vi "Init.vi"(0 "FrontPanelData in":refnum<class "EpiWrapper.lvclass">, 1 "MeasureControl":refnum<vi>, 3 "SpectrumSat":refnum<vi>, 4 "Configuration":refnum<vi>, 5 "WaferTable_Ref":refnum<vi>, 7 "error in (no error)":errorcluster, 8 "MapPositions":refnum<vi>, 9 "WaferMao":refnum<vi>, 11 "CurrentPad":refnum<vi>, 12 "Input":refnum<vi>, 13 "WaferPads":refnum<vi>, 15 "IntTime_Ref":refnum<vi>, 16 "AppPaths":refnum<vi>, 17 "INSTR_PARAM":refnum<vi>) -> (20 "FrontPanelData out":refnum<class "EpiWrapper.lvclass">, 21 "Shutdown?":bool, 27 "error out":errorcluster)   [LabVIEW 2012, in "EpiWrapper.lvclass"]
uses:
  EpiWrapper.lvclass
  Controls/Instr_Param.ctl
  Instruments/TypeDefs/SMUParam.ctl
  Controls/USB4000_Data.ctl
  Controls/WaferTable.ctl
  Controls/Config.ctl
  Controls/SelectedPads.ctl
  Controls/Pad.ctl
  Controls/MeasureControl.ctl
  Controls/PadArea.ctl
  Controls/TestData.ctl
  Controls/Measurement.ctl
  EpiWrapper.lvclass/EpiWrapper.ctl
  Instruments.lvclass
  Controls/ProbeStationId.vi
  LotData.lvclass
panel:
  # "Measure Control"
  # "Measurement Settings"
  # "Test Criteria"
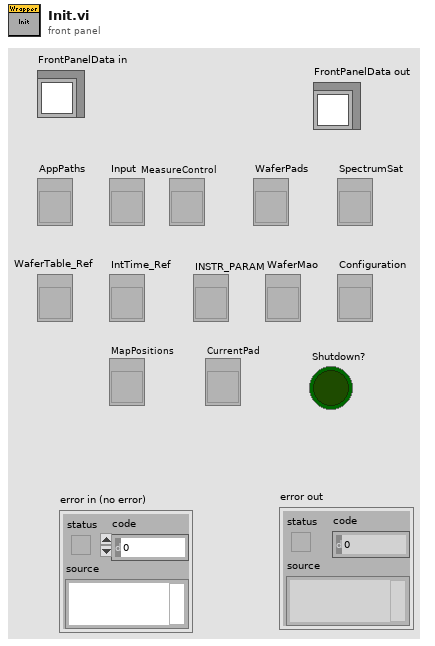
[diagram p1: front panel]
types:
  T1 = typedef "ErrorActions.ctl" = enum16{"Shutdown", "Warning", "Reset", "NoAction"}
  T2 = typedef "Config.ctl" = cluster{"IntTime":i32, "Samples":i32, "PowerMin":dbl, "KneeMin":dbl, "KneeMax":dbl, "Background Wl":dbl, "Settle Delay,ms":u32, "StationId":sgl}
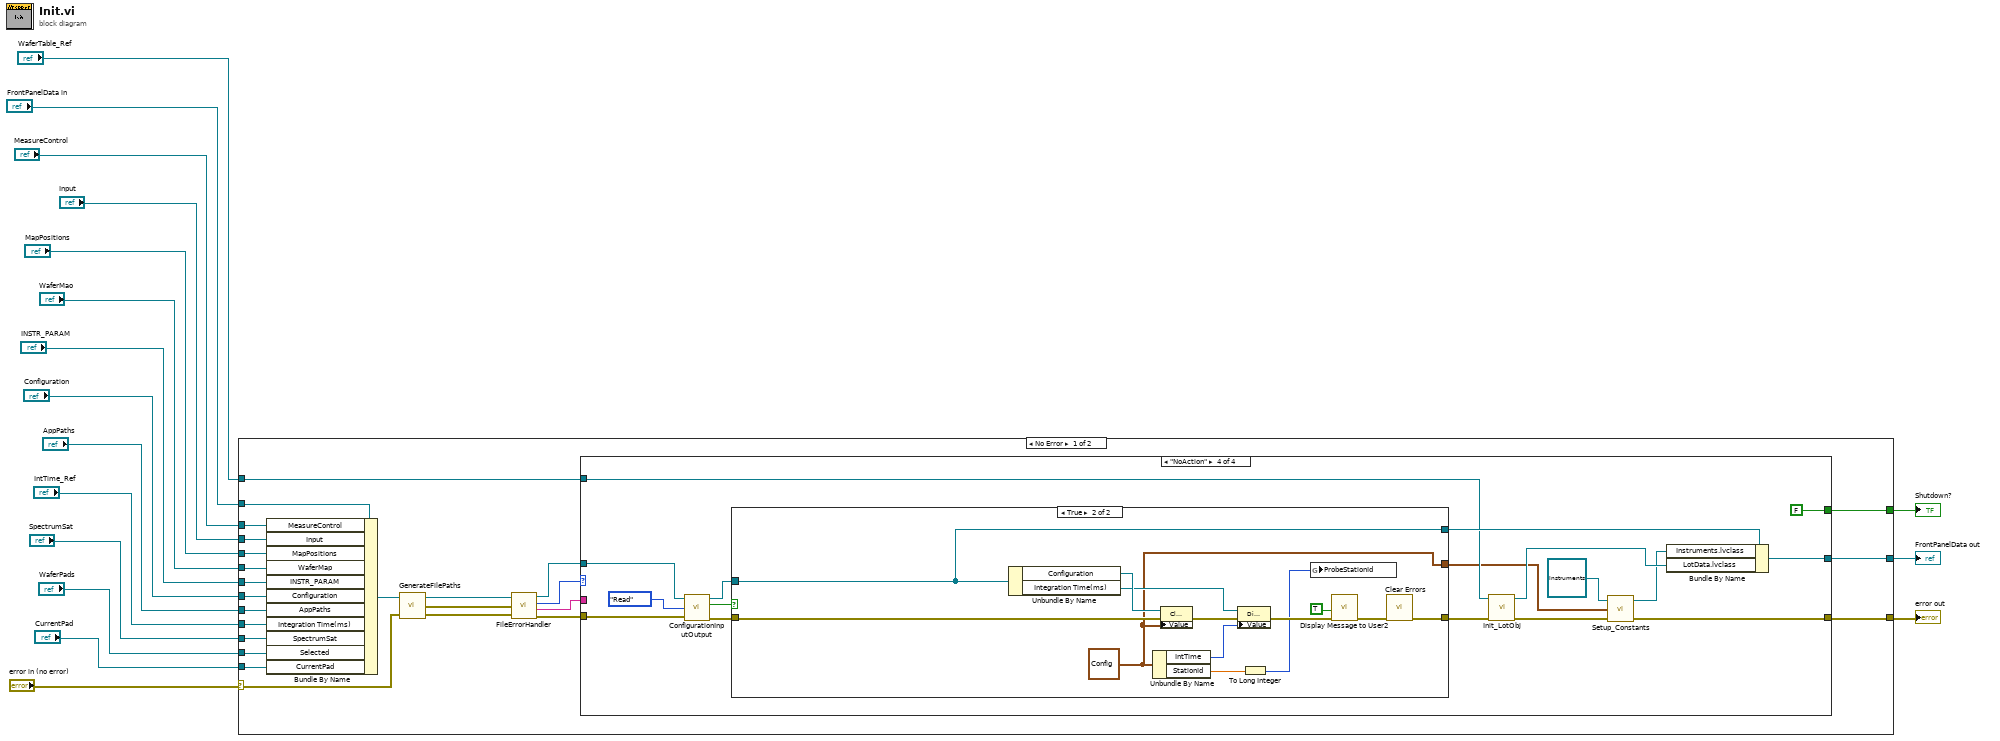
[diagram p0: block diagram]
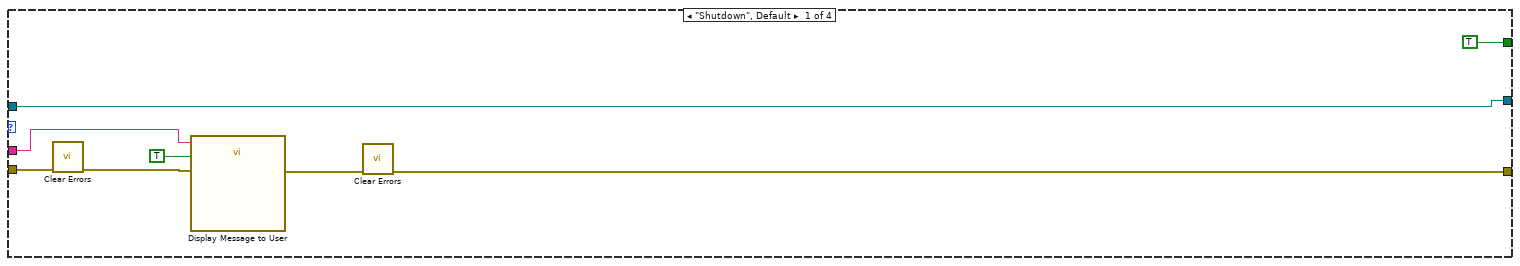
[diagram p2: hidden frame]
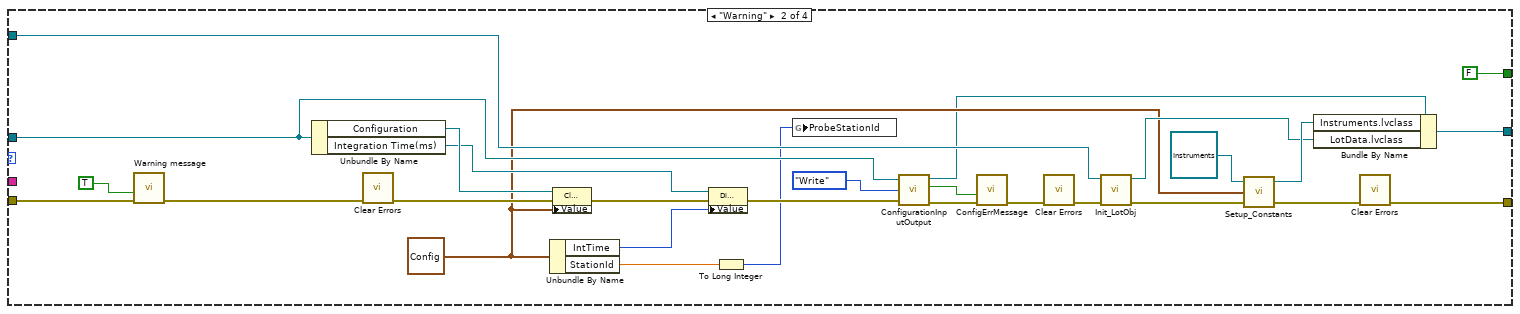
[diagram p3: hidden frame]
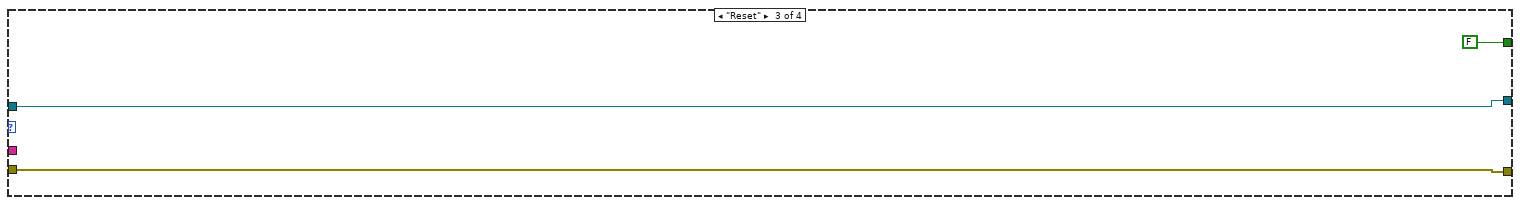
[diagram p4: hidden frame]
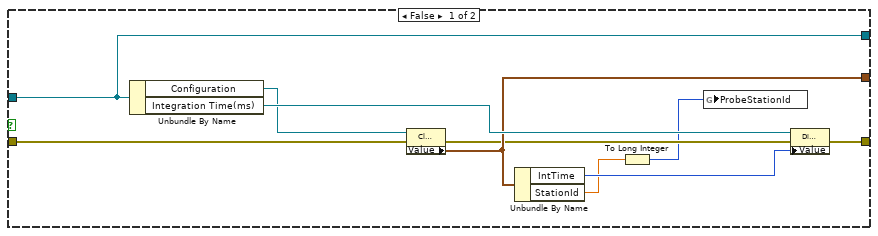
[diagram p5: hidden frame]
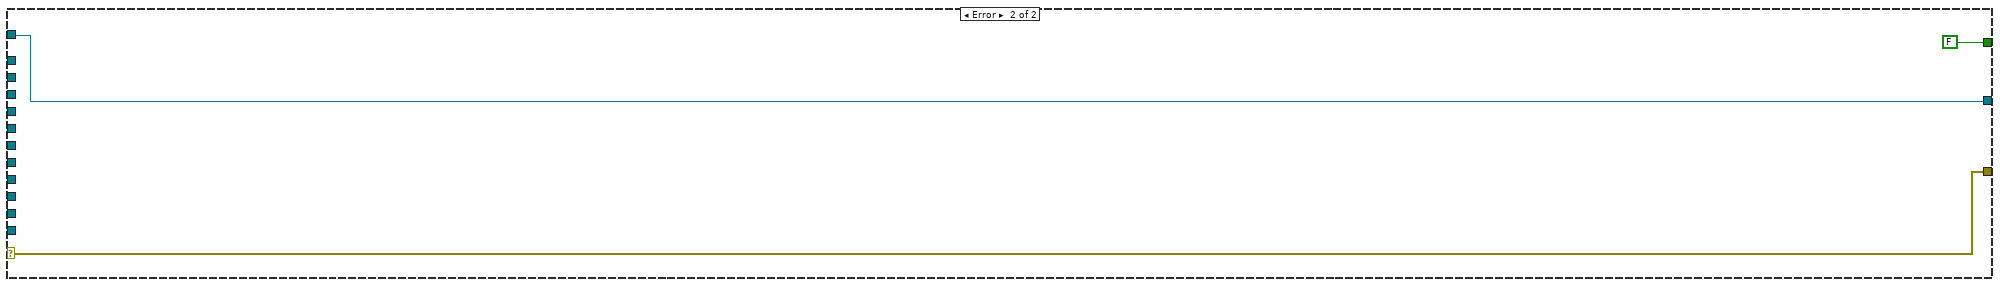
[diagram p6: hidden frame]
diagram:
  n1 = case shown="No Error" "error in (no error)" {
    selector: "error in (no error)" -> [w39 w124]
    tunnel: [w30 w124] -> w16
    tunnel: [w29 w123] -> w12
    tunnel: "FrontPanelData in" -> [w42 w123]
    tunnel: "WaferTable_Ref" -> [w32 _]
    tunnel: "Input" -> [w41 _]
    tunnel: "INSTR_PARAM" -> [w24 _]
    tunnel: "AppPaths" -> [w40 _]
    tunnel: [w28 FALSE ("Shutdown?")] -> w13
    tunnel: "IntTime_Ref" -> [w26 _]
    tunnel: "MeasureControl" -> [w25 _]
    tunnel: "Configuration" -> [w23 _]
    tunnel: "SpectrumSat" -> [w22 _]
    tunnel: "MapPositions" -> [w19 _]
    tunnel: "WaferMao" -> [w21 _]
    tunnel: "WaferPads" -> [w20 _]
    tunnel: "CurrentPad" -> [w18 _]
    frame No Error {
      n2 = Bundle By Name(cluster=w42, "MeasureControl"=w25, "Input"=w41, "MapPositions"=w19, "WaferMap"=w21, "INSTR_PARAM"=w24, "Configuration"=w23, "AppPaths"=w40, "Integration Time(ms)"=w26, "SpectrumSat"=w22, "Selected"=w20, "CurrentPad"=w18) -> (w31:refnum<class "EpiWrapper.lvclass">)
      n3 = call "GenerateFilePaths.vi"("error in (no error)"=w39, "EpiWrapper in"=w31) -> ("error out"=w37:errorcluster, "Errors"=w36:errorcluster[], "EpiWrapper out"=w38:refnum<class "EpiWrapper.lvclass">)  [unwired: 1 in]
      n4 = call-dynamic "FileErrorHandler.vi"("EpiWrapper in"=w38, "FilePathErrors"=w36, "error in (no error)"=w37) -> ("EpiWrapper out"=w33:refnum<class "EpiWrapper.lvclass">, "ErrorActions"=w35:T1, "Error Message"=w27:string, "error out"=w34:errorcluster)
      n5 = case shown="\"NoAction\"" w35 {
        tunnel: w34 -> [w47 w68 w79 w92]
        tunnel: w33 -> [w43 w61 w80 w93]
        tunnel: w32 -> [_ w73 _ w84]
        tunnel: [w45 w77 w79 w94] -> w30
        tunnel: [w43 w72 w80 w85] -> w29
        tunnel: [TRUE ("Shutdown?") FALSE ("Shutdown?") FALSE ("Shutdown?") FALSE ("Shutdown?")] -> w28
        tunnel: w27 -> [w49 _ _ _]
        frame "Shutdown", Default {
          n6 = call <vilib>:"Clear Errors.vi"("error in (no error)"=w47) -> ("error out"=w46:errorcluster)  [unwired: 6 in]
          n7 = call "Display Message to User"("error in (no error)"=w46, "Enable"=TRUE, "Message"=w49) -> ("error out"=w44:errorcluster)  [unwired: 7 in, 1 out]
          n8 = call <vilib>:"Clear Errors.vi"("error in (no error)"=w44) -> ("error out"=w45:errorcluster)  [unwired: 6 in]
        }
        frame "Warning" {
          w54 = T2 {"IntTime"=100, "Samples"=3, "PowerMin"=300.0, "KneeMin"=-20.0, "KneeMax"=20.0, "Background Wl"=0.0, "Settle Delay,ms"=0, "StationId"=0.0} ("Value")
          n9 = call "Warning message"("error in (no error)"=w68, "Enable"=TRUE) -> ("error out"=w67:errorcluster)  [unwired: 8 in, 1 out]
          n10 = Unbundle By Name(w61) -> ("Configuration"=w66:refnum<vi>, "Integration Time(ms)"=w64:refnum<vi>)
          n11 = call <vilib>:"Clear Errors.vi"("error in (no error)"=w67) -> ("error out"=w65:errorcluster)  [unwired: 6 in]
          n12 = Unbundle By Name(w54) -> ("IntTime"=w62:i32, "StationId"=w51:sgl)
          n13 = property class="Clust (strict)"(reference=w66, error in=w65, "Value"=w54) -> (error out=w63:errorcluster)  [unwired: 1 out]
          n14 = property class="DigNum (strict)"(reference=w64, error in=w63, "Value"=w62) -> (error out=w59:errorcluster)  [unwired: 1 out]
          n15 = To Long Integer(number=w51) -> (32bit integer=w52:i32)
          n16 = global write "ProbeStationId.vi" "ProbeStationId"(w52) -> ()
          n17 = call-dynamic "ConfigurationInputOutput.vi"("EpiWrapper in"=w61, "Action"=enum16{"Read", "Write"}."Write", "error in (no error)"=w59) -> ("EpiWrapper out"=w53:refnum<class "EpiWrapper.lvclass">, "error?"=w57:bool, "error out"=w56:errorcluster)  [unwired: 1 out]
          n18 = call "ConfigErrMessage"("error in (no error)"=w56, "Enable"=w57) -> ("error out"=w58:errorcluster)  [unwired: 8 in, 1 out]
          n19 = call <vilib>:"Clear Errors.vi"("error in (no error)"=w58) -> ("error out"=w55:errorcluster)  [unwired: 6 in]
          n20 = call "Init_LotObj.vi"("error in (no error)"=w55, "WaferTable_Ref"=w73) -> ("error out"=w74:errorcluster, "LotData out"=w70:refnum<class "LotData.lvclass">)  [unwired: 7 in, 1 out]
          n21 = call-dynamic "Setup_Constants.vi"("error in (no error)"=w74, "Config In"=w54, "Instruments in"=refnum<class "Instruments.lvclass"> refnum ("Instruments.lvclass")) -> ("error out"=w71:errorcluster, "Instruments out"=w76:refnum<class "Instruments.lvclass">)  [unwired: 1 in]
          n22 = Bundle By Name(cluster=w53, "Instruments.lvclass"=w76, "LotData.lvclass"=w70) -> (w72:refnum<class "EpiWrapper.lvclass">)
          n23 = call <vilib>:"Clear Errors.vi"("error in (no error)"=w71) -> ("error out"=w77:errorcluster)  [unwired: 6 in]
        }
        frame "Reset" {
        }
        frame "NoAction" {
          n24 = call-dynamic "ConfigurationInputOutput.vi"("EpiWrapper in"=w93, "Action"=enum16{"Read", "Write"}."Read", "error in (no error)"=w92) -> ("EpiWrapper out"=w90:refnum<class "EpiWrapper.lvclass">, "error?"=w87:bool, "error out"=w88:errorcluster)  [unwired: 1 out]
          n25 = case shown="True" w87 {
            tunnel: w90 -> [w105 w113]
            tunnel: [w106 w121] -> w89
            tunnel: w88 -> [w101 w119]
            tunnel: [w103 w115] -> w82
            tunnel: [w105 w113] -> w86
            frame False {
              n26 = Unbundle By Name(w105) -> ("Configuration"=w104:refnum<vi>, "Integration Time(ms)"=w108:refnum<vi>)
              n27 = property class="Clust (strict)"(reference=w104, error in=w101) -> (error out=w102:errorcluster, "Value"=w103:T2)  [unwired: 1 out]
              n28 = Unbundle By Name(w103) -> ("IntTime"=w107:i32, "StationId"=w99:sgl)
              n29 = To Long Integer(number=w99) -> (32bit integer=w100:i32)
              n30 = global write "ProbeStationId.vi" "ProbeStationId"(w100) -> ()
              n31 = property class="DigNum (strict)"(reference=w108, error in=w102, "Value"=w107) -> (error out=w106:errorcluster)  [unwired: 1 out]
            }
            frame True {
              w115 = T2 {"IntTime"=100, "Samples"=3, "PowerMin"=300.0, "KneeMin"=-20.0, "KneeMax"=20.0, "Background Wl"=0.0, "Settle Delay,ms"=0, "StationId"=0.0} ("Value")
              n32 = Unbundle By Name(w113) -> ("Configuration"=w120:refnum<vi>, "Integration Time(ms)"=w118:refnum<vi>)
              n33 = Unbundle By Name(w115) -> ("IntTime"=w117:i32, "StationId"=w110:sgl)
              n34 = property class="Clust (strict)"(reference=w120, error in=w119, "Value"=w115) -> (error out=w116:errorcluster)  [unwired: 1 out]
              n35 = property class="DigNum (strict)"(reference=w118, error in=w116, "Value"=w117) -> (error out=w112:errorcluster)  [unwired: 1 out]
              n36 = To Long Integer(number=w110) -> (32bit integer=w109:i32)
              n37 = global write "ProbeStationId.vi" "ProbeStationId"(w109) -> ()
              n38 = call "Display Message to User2"("error in (no error)"=w112, "Enable"=TRUE) -> ("error out"=w114:errorcluster)  [unwired: 8 in, 1 out]
              n39 = call <vilib>:"Clear Errors.vi"("error in (no error)"=w114) -> ("error out"=w121:errorcluster)  [unwired: 6 in]
            }
          }
          n40 = call "Init_LotObj.vi"("error in (no error)"=w89, "WaferTable_Ref"=w84) -> ("error out"=w98:errorcluster, "LotData out"=w96:refnum<class "LotData.lvclass">)  [unwired: 7 in, 1 out]
          n41 = call-dynamic "Setup_Constants.vi"("error in (no error)"=w98, "Config In"=w82, "Instruments in"=refnum<class "Instruments.lvclass"> refnum ("Instruments.lvclass")) -> ("error out"=w94:errorcluster, "Instruments out"=w95:refnum<class "Instruments.lvclass">)  [unwired: 1 in]
          n42 = Bundle By Name(cluster=w86, "Instruments.lvclass"=w95, "LotData.lvclass"=w96) -> (w85:refnum<class "EpiWrapper.lvclass">)
        }
      }
    }
    frame Error {
    }
  }
  "error out" <- w16
  "FrontPanelData out" <- w12
  "Shutdown?" <- w13
